vi "Get as U32.vi"(8 "error in (no error)":errorcluster, 10 "Name Array":string[](array[string]), 11 "JSON Scalar in":refnum<class "JSON Value.lvclass">) -> (0 "error out":errorcluster, 2 "Number":u32, 3 "JSON Scalar out":refnum<class "JSON Value.lvclass">)   [LabVIEW 2011, in "JSON Scalar.lvclass"]
doc: "Converts a <b>JSON Value</b> into a <b>Number</b>.\n\nCopyright 2012 James David Powell, Shaun Rumbell and Ton Plomp\nMore information on http://lavag.org/topic/16217-cr-json-labview"
uses:
  JSON Scalar.lvclass
  JSON Value/JSON Value.lvclass
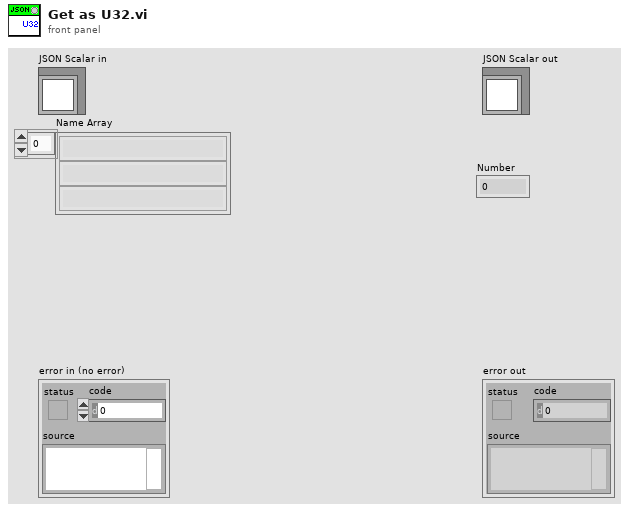
[diagram p1: front panel]
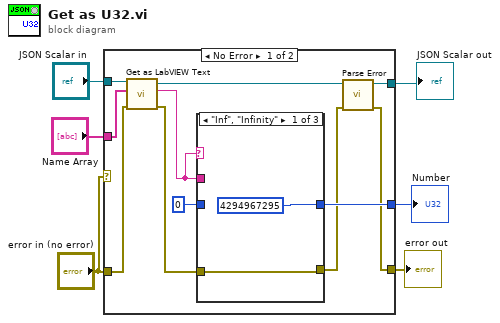
[diagram p0: block diagram]
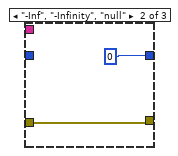
[diagram p2: hidden frame]
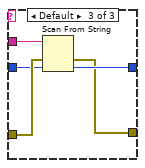
[diagram p3: hidden frame]
diagram:
  n1 = case shown="No Error" "error in (no error)" {
    tunnel: [w17 _] -> w6
    tunnel: "error in (no error)" -> [w8 w27]
    tunnel: "JSON Scalar in" -> [w15 w28]
    tunnel: [w12 w28] -> w4
    tunnel: [w10 w27] -> w3
    tunnel: "Name Array" -> [w7 _]
    frame No Error {
      n2 = call-dynamic "Get as LabVIEW Text.vi"("error in (no error)"=w8, "Name Array"=w7, "JSON Value In"=w15) -> ("error out"=w9:errorcluster, "LabVIEW Text"=w14:string, "JSON Value Out"=w13:refnum<class "JSON Value.lvclass">)  [unwired: 6 in]
      n3 = case shown="\"Inf\", \"Infinity\"" w14 {
        tunnel: [u32 4294967295 ("default value 1") u32 0 ("default value 1") w26] -> w17
        tunnel: w9 -> [w18 w20 w25]
        tunnel: [w18 w20 w24] -> w11
        tunnel: u32 0 ("default value 1") -> [_ _ w23]
        tunnel: w14 -> [_ _ w22]
        frame "Inf", "Infinity" {
        }
        frame "-Inf", "-Infinity", "null" {
        }
        frame Default {
          n4 = Scan From String(input string=w22, error in=w25, default 1=w23) -> (error out=w24:errorcluster, output 1=w26:u32)  [unwired: 2 in, 2 out]
        }
      }
      n5 = call-dynamic "Parse Error.vi"("error in (no error)"=w11, "JSON Value in"=w13) -> ("error out"=w10:errorcluster, "JSON Value out"=w12:refnum<class "JSON Value.lvclass">)  [unwired: 8 in]
    }
    frame Error {
    }
  }
  "error out" <- w3
  "JSON Scalar out" <- w4
  "Number" <- w6
